vi "AnalogInput-Waveform.vi"() -> ()   [LabVIEW 2017]
uses:
  <vilib>/DAQmx/read.llb/DAQmx Read (Analog Wfm 1Chan NSamp).vi
  <vilib>/DAQmx/create/channels.llb/DAQmx Create Channel (AI-Voltage-Basic).vi
  <vilib>/DAQmx/configure/timing.llb/DAQmx Timing (Sample Clock).vi
  <vilib>/DAQmx/miscellaneous.llb/DAQmx Fill In Error Info.vi
  <vilib>/Waveform/WDTOps.llb/WDT Append Waveforms DBL.vi
panel:
  out "Loop Time in ms":u32
  in  "Boolean":bool
  in  "number of samples per channel":i32=2000
  out "Waveform Graph":waveform(dbl)(graph)
  out "error out":errorcluster
  in  "rate":dbl=1000.0 format="%0.2f"
  in  "physical channels":tag
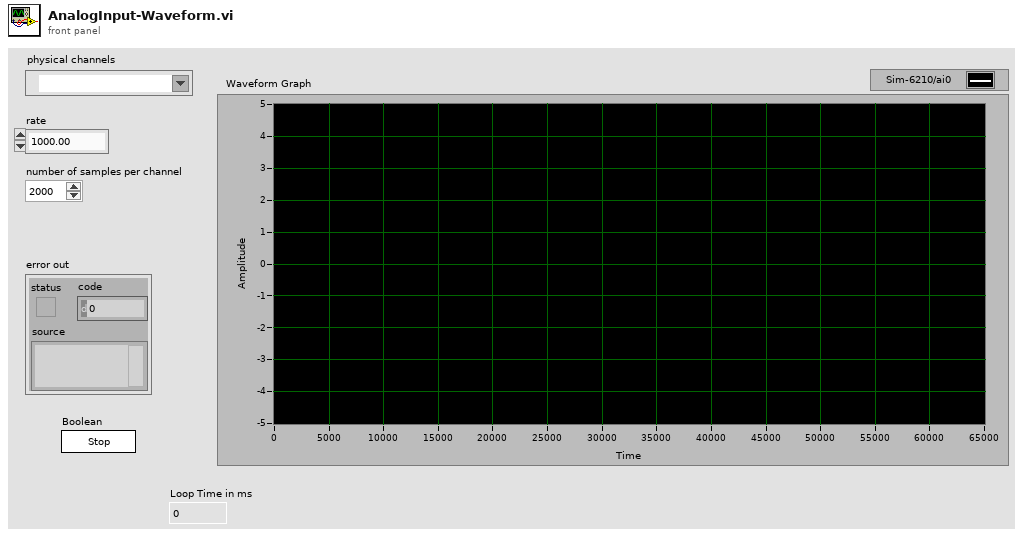
[diagram p1: front panel]
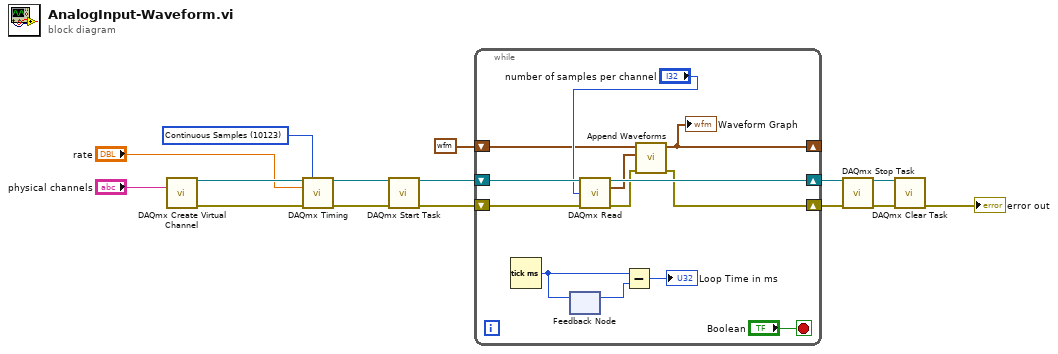
[diagram p0: block diagram]
diagram:
  w11 = 10123 items=["Finite Samples"=10178, "Continuous Samples"=10123, "Hardware Timed Single Point"=12522] ("sample mode")
  n1 = call-poly <vilib>:"DAQmx Create Virtual Channel.vi"("physical channels"="physical channels") -> ("task out"=w14:refnum<k21>, "error out"=w13:errorcluster)  [unwired: 13 in]
  n2 = call-poly <vilib>:"DAQmx Timing.vi"("task/channels in"=w14, "sample mode"=w11, "rate"="rate", "error in"=w13) -> ("task out"=w3:refnum<k21>, "error out"=w10:errorcluster)  [unwired: 10 in]
  n3 = call <vilib>:"DAQmx Start Task.vi"("task/channels in"=w3, "error in"=w10) -> ("task out"=w2:refnum<k21>, "error out"=w4:errorcluster)  [unwired: 12 in]
  n4 = while {
    shift-right: [w26] -> w6
    shift-left: w2 -> [w28]
    shift-right: [w16] -> w9
    shift-left: w4 -> [w27]
    shift-right: [w19] -> _
    shift-left: waveform(dbl) {"t0"=timestamp(0 s since 1904-01-01), "dt"=1.0, "Y"=[]} ("waveform out") -> [w20]
    stop <- "Boolean" stop-if-true
    n5 = Tick Count (ms)() -> (millisecond timer value=w24:u32)
    n6 = feedback-in #1(w24) -> ()
    n7 = feedback #1() -> (w23:u32)  [unwired: 1 in]
    n8 = call-poly <vilib>:"DAQmx Read.vi"("task/channels in"=w28, "number of samples per channel"="number of samples per channel", "error in"=w27) -> ("task out"=w26:refnum<k21>, "data"=w18:waveform(dbl), "error out"=w17:errorcluster)  [unwired: 10 in]
    n9 = Subtract(x=w24, y=w23) -> (x-y=→"Loop Time in ms":u32)
    n10 = call-poly <vilib>:"Append Waveforms.vi"("error in (no error)"=w17, "waveform B"=w18, "waveform A"=w20) -> ("error out"=w16:errorcluster, "waveform out"=w19:waveform(dbl))  [unwired: 7 in]
    "Waveform Graph" <- w19
  }
  n11 = call <vilib>:"DAQmx Stop Task.vi"("task/channels in"=w6, "error in"=w9) -> ("task out"=w5:refnum<k21>, "error out"=w7:errorcluster)  [unwired: 12 in]
  n12 = call <vilib>:"DAQmx Clear Task.vi"("task in"=w5, "error in"=w7) -> ("error out"=→"error out":errorcluster)  [unwired: 13 in]
